vi "CalGas berechnen.vi"(6 "Aktion":enum16{"lesen", "berechnen"}(ring), 7 "Index":i32, 10 "Sollwerte":T2 {"Sollwert 6" format="%#_10f"; "Sollwert 5" format="%#_10f"; "Sollwert 4" format="%#_10f"; "Sollwert 3" format="%#_10f"; "Sollwert 2" format="%#_10f"; "Sollwert 1" format="%#_10f"}, 11 "Istwert":sgl[](array[numeric])) -> (1 "Ist Abweichung":sgl[](array[numeric]), 2 "Index":i32, 3 "Ist\nAbweichung":T1 {"Abweichung 6" format="%#_5g"; "Abweichung 5" format="%#_5g"; "Abweichung 4" format="%#_5g"; "Abweichung 3" format="%#_5g"; "Abweichung 2" format="%#_5g"; "Abweichung 1" format="%#_5g"})   [LabVIEW 2020, in "Erweiterte Konfig.lvlib" / "CG-Check Konfig.lvlib"]
uses:
  CG-Check Konfig.lvlib
  Aktion_CG-Check.ctl
panel:
  in  "Ist\nAbweichung":T1 {"Abweichung 6" format="%#_5g"; "Abweichung 5" format="%#_5g"; "Abweichung 4" format="%#_5g"; "Abweichung 3" format="%#_5g"; "Abweichung 2" format="%#_5g"; "Abweichung 1" format="%#_5g"}
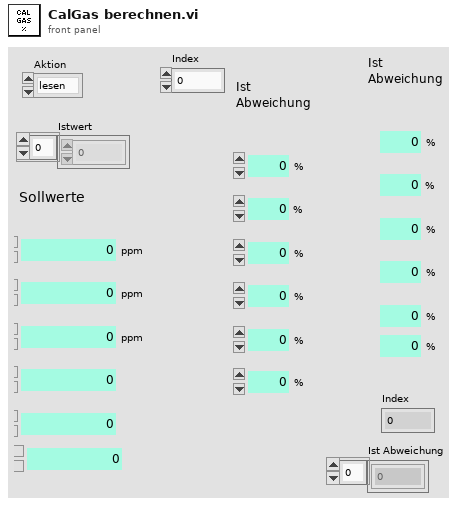
[diagram p1: front panel]
types:
  T1 = cluster{"Abweichung 1":sgl, "Abweichung 2":sgl, "Abweichung 3":sgl, "Abweichung 4":sgl, "Abweichung 5":sgl, "Abweichung 6":sgl}
  T2 = cluster{"Sollwert 1":sgl, "Sollwert 2":sgl, "Sollwert 3":sgl, "Sollwert 4":sgl, "Sollwert 5":sgl, "Sollwert 6":sgl}
  T3 = typedef "Erweiterte Konfig.lvlib/CG-Check Konfig.lvlib/Aktion_CG-Check.ctl" = enum16{"lesen", "schreiben", "laden", "Komponente", "Aktive?", "speichern"}
  T4 = cluster{"[0]":sgl, "[1]":sgl, "[2]":sgl, "[3]":sgl, "[4]":sgl, "[5]":sgl, "[6]":sgl, "[7]":sgl, "[8]":sgl}
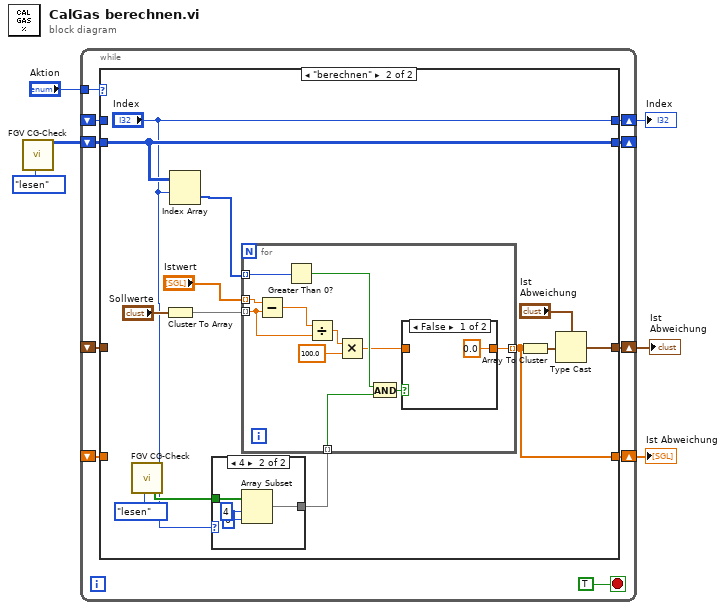
[diagram p0: block diagram]
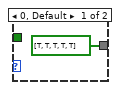
[diagram p3: hidden frame]
diagram:
  n1 = call "FGV CG-Check.vi"("Aktion"=Aktion_CG-Check."lesen") -> ("Komponenten"=w3:u16[][])  [unwired: 11 in, 7 out]
  n2 = while {
    tunnel: "Aktion" -> [w15]
    shift-right: [w14] -> w5
    shift-left: _ -> [w13]
    shift-right: [w12] -> _
    shift-left: w3 -> [w11]
    shift-right: [w10] -> w2
    shift-left: _ -> [w9]
    shift-right: [w8] -> w1
    shift-left: _ -> [w7]
    stop <- TRUE stop-if-true
    n3 = case shown="\"berechnen\"" w15 {
      tunnel: [w20 w28] -> w14
      tunnel: w13 -> [w20 _]
      tunnel: w11 -> [w19 w27]
      tunnel: [w19 w27] -> w12
      tunnel: [w18 "Index"] -> w10
      tunnel: w9 -> [w18 _]
      tunnel: [w17 w25] -> w8
      tunnel: w7 -> [w17 _]
      frame "lesen", Default {
      }
      frame "berechnen" {
        n4 = call "FGV CG-Check.vi"("Aktion"=Aktion_CG-Check."lesen") -> ("Aktive?"=w24:bool[])  [unwired: 11 in, 7 out]
        n5 = Cluster To Array(cluster="Sollwerte") -> (array=w31:sgl[])
        n6 = Index Array ("Istwert")(array=w27, index (row)="Index") -> (element=w26:u16[])  [unwired: 1 in]
        n7 = case shown="4" "Index" {
          tunnel: w24 -> [_ w38]
          tunnel: [bool[] [TRUE, TRUE, TRUE, TRUE, TRUE] w37] -> w21
          frame 0, Default {
          }
          frame 4 {
            n8 = Array Subset(array=w38, index=4 ("Index"), length=6 ("Länge")) -> (w37:bool[])
          }
        }
        n9 = for {
          tunnel: "Istwert" -> [w49] mode=indexing
          tunnel: w31 -> [w44] mode=indexing
          tunnel: [w40] -> w25 mode=indexing
          tunnel: w26 -> [w45] mode=indexing
          tunnel: w21 -> [w43] mode=indexing
          n10 = Subtract(x=w49, y=w44) -> (x-y=w48:sgl)
          n11 = Greater Than 0?(x=w45) -> (x > 0?=w42:bool)
          n12 = Divide(x=w48, y=w44) -> (x/y=w47:sgl)
          n13 = Multiply(x=w47, y=sgl 100.0) -> (x*y=w39:sgl)
          n14 = And(x=w42, y=w43) -> (x .and. y?=w41:bool)
          n15 = case shown="False" w41 {
            tunnel: [sgl 0.0 w51] -> w40
            tunnel: w39 -> [_ w51]
            frame False {
            }
            frame True {
            }
          }
        }
        n16 = Array To Cluster(array=w25) -> (cluster=w29:T4)
        n17 = Type Cast(type="Ist\nAbweichung", x=w29) -> (*(type *) &x=w28:T1)
      }
    }
  }
  "Ist\nAbweichung" <- w5
  "Index" <- w2
  "Ist Abweichung" <- w1
